vi "UART Write.vi"(4 "write buffer":string, 5 "error in (no error)":errorcluster, 6 "Add Return":bool=TRUE, 7 "Write Delay (s)":dbl caption="Delay Time (s)", 8 "VISA Resource In":refnum<visa-resource-name>="COM1") -> (0 "error out":errorcluster, 3 "VISA Resource Out":refnum<visa-resource-name>)   [LabVIEW 2015]
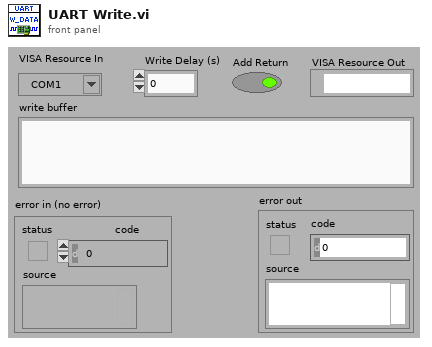
[diagram p1: front panel]
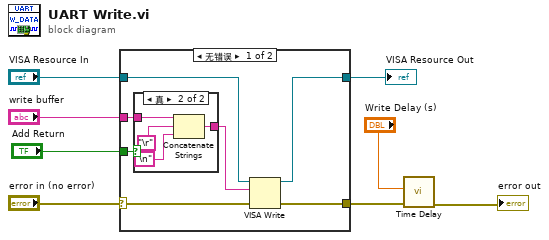
[diagram p0: block diagram]
diagram:
  n1 = case shown="无错误" "error in (no error)" {
    selector: "error in (no error)" -> [w10 w21]
    tunnel: "VISA Resource In" -> [w15 w22]
    tunnel: [w14 w21] -> w4
    tunnel: [w13 w22] -> w7
    tunnel: "write buffer" -> [w12 _]
    tunnel: "Add Return" -> [w9 _]
    frame No Error {
      n2 = case shown="真" w9 {
        tunnel: w12 -> [w16 w20]
        tunnel: [w16 w19] -> w11
        frame False {
        }
        frame True {
          n3 = Concatenate Strings(w20, "\r", "\n") -> (w19:string)
        }
      }
      n4 = VISA Write(VISA resource name=w15, write buffer=w11, error in (no error)=w10) -> (VISA resource name out=w13:refnum<visa-resource-name>, error out=w14:errorcluster)  [unwired: 1 out]
    }
    frame Error {
    }
  }
  "VISA Resource Out" <- w7
  n5 = call "Time Delay"("error in (no error)"=w4, "Delay Time (s)"="Write Delay (s)") -> ("error out"=→"error out":errorcluster)  [unwired: 9 in]
